vi "Simple Put.vi"   [LabVIEW 2017, in "NI_WebDAV.lvlib"]
doc: "Uploads a file or multiple files to a remote WebDAV server or target. You must manually select the polymorphic instance you want to use."
uses:
  <vilib>/WebDAVClient/NI_WebDAV.lvlib
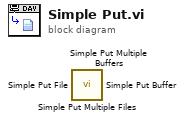
[diagram p0: block diagram]
diagram:
  n1 = call <vilib>:"Simple Put Multiple Files.vi"() -> ()  [unwired: 15 in, 1 out]
  n2 = call <vilib>:"Simple Put Multiple Buffers.vi"() -> ()  [unwired: 15 in, 1 out]
  n3 = call <vilib>:"Simple Put File.vi"() -> ()  [unwired: 14 in, 2 out]
  n4 = call <vilib>:"Simple Put Buffer.vi"() -> ()  [unwired: 15 in, 1 out]
